vi "save_tdms.vi"(6 "filename":string, 7 "waveform signal":waveform(dbl)[](array[waveform]), 8 "error in (no error)":errorcluster, 9 "Array":T1(array[cluster]), 10 "Numeric":i32, 11 "Folder with vibration":path) -> (0 "error out":errorcluster)   [LabVIEW 2025]
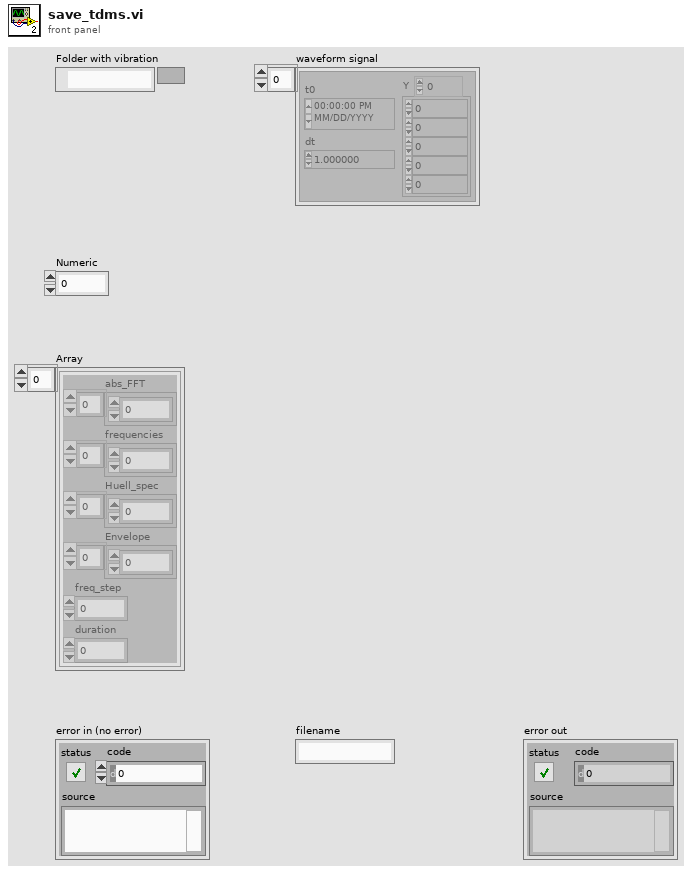
[diagram p1: front panel]
types:
  T1 = cluster{"abs_FFT":dbl[], "frequencies":dbl[], "Huell_spec":dbl[], "Envelope":dbl[], "freq_step":dbl, "duration":dbl}[]
  T2 = enum16{"open", "open or create", "create or replace", "create", "open (read-only)"}
  T3 = cluster{"abs_FFT":dbl[], "frequencies":dbl[], "Huell_spec":dbl[], "Envelope":dbl[], "freq_step":dbl, "duration":dbl}
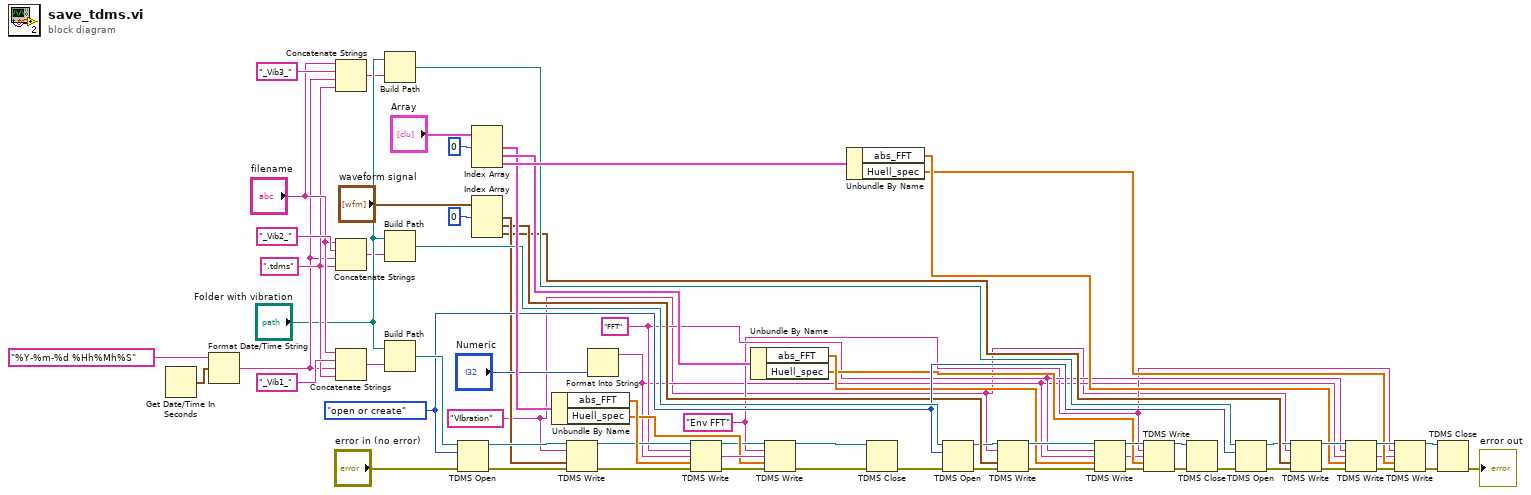
[diagram p0: block diagram]
diagram:
  w43 = ".tdms" ("String")
  w36 = T2."open or create" ("Operation (0:open)")
  w13 = "Env FFT" ("Gruppenname (Eingang, Unbenannt)")
  w14 = "FFT" ("Gruppenname (Eingang, Unbenannt)")
  w9 = "VIbration" ("Gruppenname (Eingang, Unbenannt)")
  n1 = Get Date/Time In Seconds() -> (seconds since 1Jan1904=w48:timestamp)
  n2 = Format Date/Time String(time format string (%c)="%Y-%m-%d %Hh%Mh%S" ("Zeitformatierungs-String (%c)"), seconds (now)=w48) -> (date/time string=w42:string)  [unwired: 1 in]
  n3 = Concatenate Strings("filename", "_Vib3_" ("string"), w42, w43) -> (w39:string)
  n4 = Concatenate Strings("filename", "_Vib2_" ("string"), w42, w43) -> (w40:string)
  n5 = Concatenate Strings("filename", "_Vib1_" ("string"), w42, w43) -> (w55:string)
  n6 = Build Path(base path="Folder with vibration", name or relative path=w39) -> (appended path=w37:path)
  n7 = Build Path(base path="Folder with vibration", name or relative path=w40) -> (appended path=w38:path)
  n8 = Build Path(base path="Folder with vibration", name or relative path=w55) -> (appended path=w56:path)
  n9 = TDMS Open(8:"error in (no error)", 10:w36, 11:w56) -> (0:w58:errorcluster, 3:w53:refnum<k34>)  [unwired: 4 in]
  n10 = Index Array(array="Array", index #1=0 ("index")) -> (element #1=w62:T3, element #2=w63:T3, element #3=w64:T3)  [unwired: 2 in]
  n11 = Index Array(array="waveform signal", index #1=0 ("index")) -> (element #1=w33:waveform(dbl), element #2=w32:waveform(dbl), element #3=w31:waveform(dbl))  [unwired: 2 in]
  n12 = Unbundle By Name(w62) -> ("abs_FFT"=w68:dbl[], "Huell_spec"=w65:dbl[])
  n13 = TDMS Write(0:w53, 5:w9, 9:w33, 11:w58) -> (4:w49:refnum<k34>, 15:w50:errorcluster)  [unwired: 2 in, 2 out]
  n14 = Format Into String("Numeric") -> (resulting string=w12:string)  [unwired: 3 in, 1 out]
  n15 = TDMS Write(0:w49, 5:w14, 7:w12, 9:w68, 11:w50) -> (4:w52:refnum<k34>, 8:w66:string, 15:w51:errorcluster)  [unwired: 1 in, 1 out]
  n16 = Unbundle By Name(w63) -> ("abs_FFT"=w18:dbl[], "Huell_spec"=w17:dbl[])
  n17 = TDMS Write(0:w52, 5:w13, 7:w66, 9:w65, 11:w51) -> (4:w8:refnum<k34>, 15:w7:errorcluster)  [unwired: 1 in, 2 out]
  n18 = Unbundle By Name(w64) -> ("abs_FFT"=w16:dbl[], "Huell_spec"=w15:dbl[])
  n19 = TDMS Close(8:w7, 11:w8) -> (0:w6:errorcluster)  [unwired: 1 out]
  n20 = TDMS Open(8:w6, 10:w36, 11:w38) -> (0:w28:errorcluster, 3:w27:refnum<k34>)  [unwired: 4 in]
  n21 = TDMS Write(0:w27, 5:w9, 9:w32, 11:w28) -> (4:w24:refnum<k34>, 15:w26:errorcluster)  [unwired: 2 in, 2 out]
  n22 = TDMS Write(0:w24, 5:w14, 7:w12, 9:w18, 11:w26) -> (4:w23:refnum<k34>, 8:w11:string, 15:w25:errorcluster)  [unwired: 1 in, 1 out]
  n23 = TDMS Write(0:w23, 5:w13, 7:w11, 9:w17, 11:w25) -> (4:w5:refnum<k34>, 15:w4:errorcluster)  [unwired: 1 in, 2 out]
  n24 = TDMS Close(8:w4, 11:w5) -> (0:w3:errorcluster)  [unwired: 1 out]
  n25 = TDMS Open(8:w3, 10:w36, 11:w37) -> (0:w29:errorcluster, 3:w30:refnum<k34>)  [unwired: 4 in]
  n26 = TDMS Write(0:w30, 5:w9, 9:w31, 11:w29) -> (4:w22:refnum<k34>, 15:w21:errorcluster)  [unwired: 2 in, 2 out]
  n27 = TDMS Write(0:w22, 5:w14, 7:w12, 9:w16, 11:w21) -> (4:w20:refnum<k34>, 8:w10:string, 15:w19:errorcluster)  [unwired: 1 in, 1 out]
  n28 = TDMS Write(0:w20, 5:w13, 7:w10, 9:w15, 11:w19) -> (4:w1:refnum<k34>, 15:w2:errorcluster)  [unwired: 1 in, 2 out]
  n29 = TDMS Close(8:w2, 11:w1) -> (0:→"error out":errorcluster)  [unwired: 1 out]
